vi "Copy Pixmap to Image (Greyscale with Mask Output).vi"(8 "error in (no error)":errorcluster, 9 "Greyscale Image Mask":T1, 10 "Greyscale Image Destination":T1, 11 "Pixmap Image Data":T2) -> (0 "error out":errorcluster, 2 "Greyscale Image Mask (duplicate)":T1, 3 "Greyscale Image Destination (duplicate)":T1)   [LabVIEW 2020, in "g_ar_toolkit.image.lvlib"]
uses:
  g_ar_toolkit.image.lvlib
  Greyscale Image.ctl
  <vilib>/picture/picture.llb/imagedata.ctl
  3b7a14f1-ed28-461e-8305-e3c68bcd5d6e.vi
  FixPixmap.vi
  Default8bitColourMap.vi
  <vilib>/Utility/error.llb/Error Cluster From Error Code.vi
  g_ar_toolkit.common/Module Path.vi
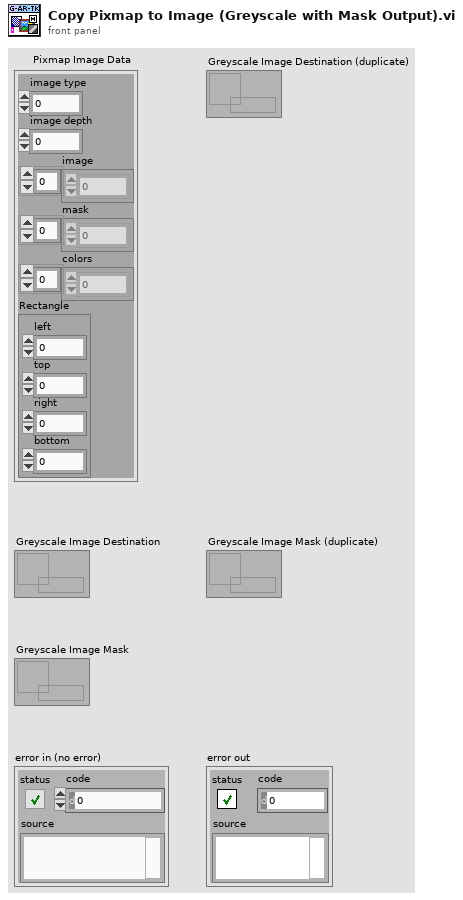
[diagram p1: front panel]
types:
  T1 = typedef "g_ar_toolkit.image.lvlib/Greyscale Image.ctl" = refnum<data-value>
  T2 = typedef "imagedata.ctl" = cluster{"image type":i32, "image depth":i32, "image":u8[], "mask":u8[], "colors":u32[], "Rectangle":cluster{"left":i16, "top":i16, "right":i16, "bottom":i16}}
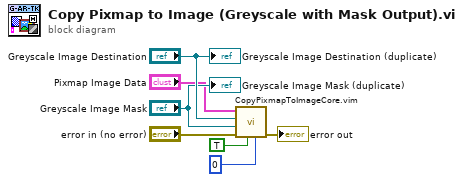
[diagram p0: block diagram]
diagram:
  n1 = call "CopyPixmapToImageCore.vim"("Background Value"=u32 0, "Has Mask"=TRUE, "error in (no error)"="error in (no error)", "Mask Image"="Greyscale Image Mask", "Source Image"="Greyscale Image Destination", "image data"="Pixmap Image Data") -> ("error out"=→"error out":errorcluster)  [unwired: 5 in]
  "Greyscale Image Destination (duplicate)" <- "Greyscale Image Destination"
  "Greyscale Image Mask (duplicate)" <- "Greyscale Image Mask"
